vi "cook.vi"(8 "error in (no error)":errorcluster, 11 "Reheat in":refnum<class "Reheat.lvclass">) -> (0 "error out":errorcluster, 3 "Reheat out":refnum<class "Reheat.lvclass">)   [LabVIEW 2010, in "CookBehaviors.lvlib" / "Reheat.lvclass"]
uses:
  Reheat.lvclass
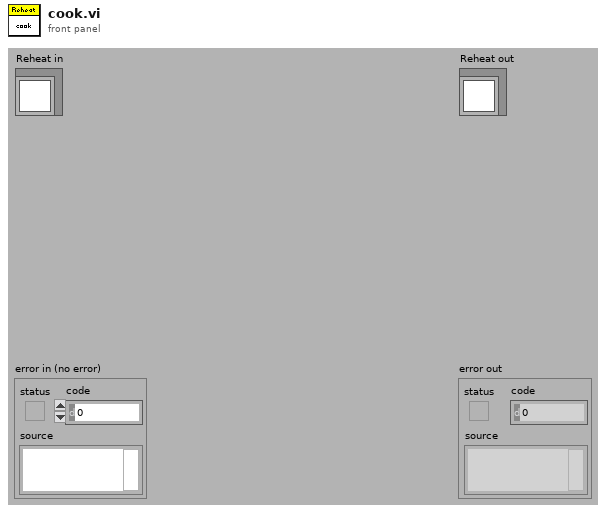
[diagram p1: front panel]
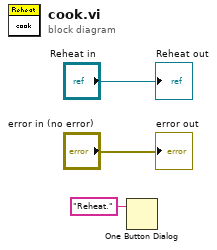
[diagram p0: block diagram]
diagram:
  n1 = One Button Dialog(message="Reheat.") -> ()  [unwired: 1 in, 1 out]
  "error out" <- "error in (no error)"
  "Reheat out" <- "Reheat in"
